vi "Point Data Updated.vi"(8 "error in (no error)":errorcluster, 9 "Data":variant, 10 "Task-Point Ident":string, 11 "ISeries UI Actor in":refnum<class "ISeries UI Actor.lvclass">) -> (0 "error out":errorcluster, 3 "ISeries UI Actor out":refnum<class "ISeries UI Actor.lvclass">)   [LabVIEW 2024, in "ISeries UI Actor.lvlib" / "ISeries UI Actor.lvclass"]
uses:
  ISeries UI Actor.lvclass
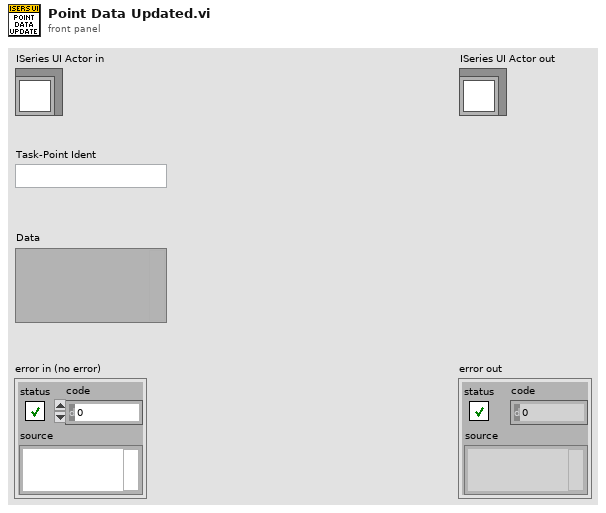
[diagram p1: front panel]
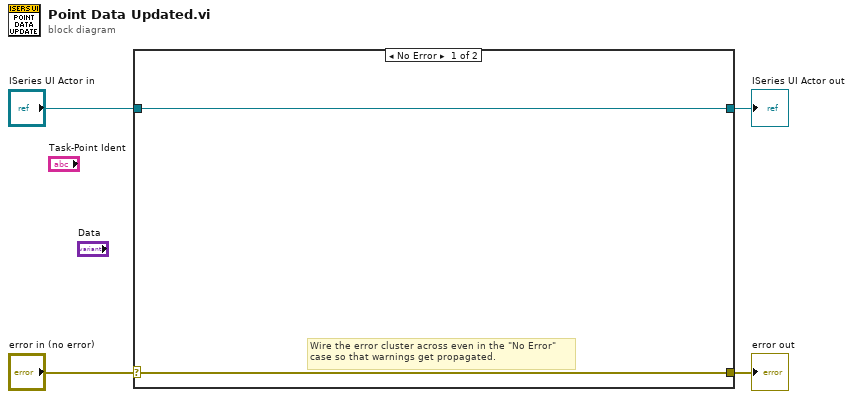
[diagram p0: block diagram]
diagram:
  n1 = case shown="No Error" "error in (no error)" {
    selector: "error in (no error)" -> [w5 w8]
    tunnel: [w5 w8] -> w3
    tunnel: [w6 w7] -> w1
    tunnel: "ISeries UI Actor in" -> [w6 w7]
    frame No Error {
      # "Wire the error cluster across even in the \"No Error\"\ncase so that warnings get propagated."
    }
    frame Error {
    }
  }
  "error out" <- w3
  "ISeries UI Actor out" <- w1
